vi "Register SGL.vi"(10 "Value":sgl, 11 "Register":T1) -> (3 "Data":u8[](array[numeric]))   [LabVIEW 2020, in "Rover.lvlib" / "Rover.lvclass"]
uses:
  Rover.lvclass
  I2C Register.ctl
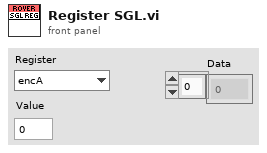
[diagram p1: front panel]
types:
  T1 = typedef "Rover.lvlib/Rover.lvclass/I2C Register.ctl" = enum8{"encA", "encB", "ticksPerUnit", "width", "flags", "velP", "velI", "velD", "velMin", "velMax", "poseX", "poseY", "poseA", "cmdDrive", "cmdTurn", "velocity", "turn", "velL", "velR", "run", "outL", "outR", "outDeadband"}
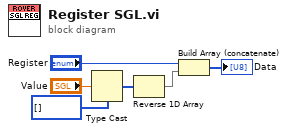
[diagram p0: block diagram]
diagram:
  n1 = Type Cast(type=u8[] [], x="Value") -> (*(type *) &x=w5:u8[])
  n2 = Reverse 1D Array(array=w5) -> (reversed array=w4:u8[])
  n3 = Build Array (concatenate)("Register", w4) -> (→"Data":u8[])
